vi "DDS.vi"() -> ()   [LabVIEW 2021]
uses:
  <vilib>/RTI DDS Toolkit/Types/RTI DDS Advanced Writer Configuration.ctl
  <vilib>/RTI DDS Toolkit/Types/RTI DDS Advanced Reader Configuration.ctl
  <vilib>/RTI DDS Toolkit/VIs/AdvancedCreateReader_NumI32.vi
  <vilib>/RTI DDS Toolkit/VIs/AdvancedCreateWriter_NumI32.vi
  <vilib>/RTI DDS Toolkit/VIs/Read_NumI32.vi
  <vilib>/RTI DDS Toolkit/VIs/Write_NumI32.vi
  <vilib>/RTI DDS Toolkit/Library/LVDDS_library.lvlib
panel:
  out "Control Time (ms)":i32
  out "Real Time (ms)":u32
  in  "Advanced Reader Configuration":T1={"typeName"="std_msgs::msg::dds_::Int32_", "keyName"="", "domainParticipantQoSProfile"="", "dataReaderQoSProfile"="", "forceArrayMapping?"=FALSE, "forceExclusiveReader?"=FALSE, "forceRead? (only ExclusiveReader)"=FALSE, "forceUnboundedString?"=FALSE}
  in  "Advanced Writer Configuration":T2={"typeName"="std_msgs::msg::dds_::Int32_", "keyName"="", "domainParticipantQoSProfile"="", "dataWriterQoSProfile"="", "forceArrayMapping?"=FALSE, "forceUnboundedString?"=FALSE}
  in  "stop":bool
  # "DDS"
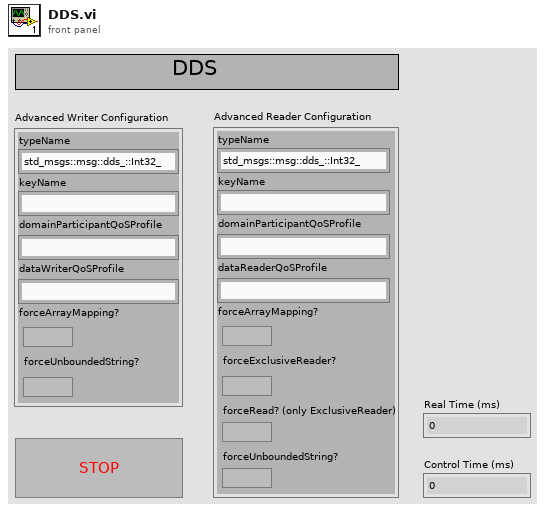
[diagram p1: front panel]
types:
  T1 = typedef "LVDDS_library.lvlib/RTI DDS Advanced Reader Configuration.ctl" = cluster{"typeName":string, "keyName":string, "domainParticipantQoSProfile":string, "dataReaderQoSProfile":string, "forceArrayMapping?":bool, "forceExclusiveReader?":bool, "forceRead? (only ExclusiveReader)":bool, "forceUnboundedString?":bool}
  T2 = typedef "LVDDS_library.lvlib/RTI DDS Advanced Writer Configuration.ctl" = cluster{"typeName":string, "keyName":string, "domainParticipantQoSProfile":string, "dataWriterQoSProfile":string, "forceArrayMapping?":bool, "forceUnboundedString?":bool}
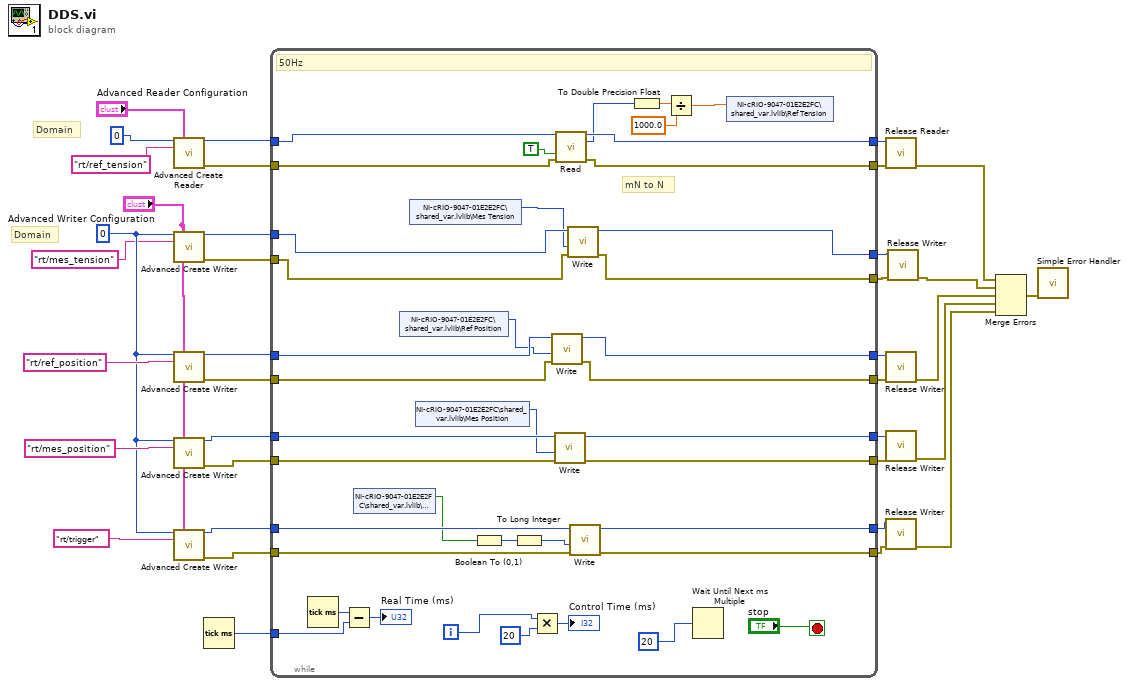
[diagram p0: block diagram]
diagram:
  w4 = u32 0 ("Domain Id")
  # "Domain"
  # "Domain"
  n1 = call-poly <vilib>:"Advanced Create Reader.vi"("Domain Id"=u32 0, "Advanced Reader Configuration"="Advanced Reader Configuration", "Topic Name"="rt/ref_tension") -> ("DDS Object Ref"=w20:u64, "error out"=w21:errorcluster)  [unwired: 11 in]
  n2 = call-poly <vilib>:"Advanced Create Writer.vi"("Domain Id"=w4, "Advanced Writer Configuration"="Advanced Writer Configuration", "Topic Name"="rt/mes_tension") -> ("DDS Object Ref"=w9:u64, "error out"=w8:errorcluster)  [unwired: 11 in]
  n3 = call-poly <vilib>:"Advanced Create Writer.vi"("Domain Id"=w4, "Advanced Writer Configuration"="Advanced Writer Configuration", "Topic Name"="rt/ref_position") -> ("DDS Object Ref"=w15:u64, "error out"=w16:errorcluster)  [unwired: 11 in]
  n4 = call-poly <vilib>:"Advanced Create Writer.vi"("Domain Id"=w4, "Advanced Writer Configuration"="Advanced Writer Configuration", "Topic Name"="rt/mes_position") -> ("DDS Object Ref"=w35:u64, "error out"=w34:errorcluster)  [unwired: 11 in]
  n5 = call-poly <vilib>:"Advanced Create Writer.vi"("Domain Id"=w4, "Advanced Writer Configuration"="Advanced Writer Configuration", "Topic Name"="rt/trigger") -> ("DDS Object Ref"=w27:u64, "error out"=w28:errorcluster)  [unwired: 11 in]
  n6 = Tick Count (ms)() -> (millisecond timer value=w10:u32)
  n7 = while {
    tunnel: w10 -> [w51]
    tunnel: w27 -> [w70]
    tunnel: [w69] -> w26
    tunnel: w28 -> [w71]
    tunnel: [w68] -> w25
    tunnel: w34 -> [w74]
    tunnel: [w72] -> w32
    tunnel: w35 -> [w75]
    tunnel: [w73] -> w33
    tunnel: w16 -> [w63]
    tunnel: [w61] -> w14
    tunnel: w15 -> [w62]
    tunnel: [w60] -> w13
    tunnel: w9 -> [w46]
    tunnel: w8 -> [w45]
    tunnel: [w44] -> w7
    tunnel: [w43] -> w6
    tunnel: w21 -> [w67]
    tunnel: [w64] -> w18
    tunnel: w20 -> [w66]
    tunnel: [w65] -> w19
    i -> [w50]
    stop <- "stop" stop-if-true
    # "mN to N"
    # "50Hz"
    n8 = Tick Count (ms)() -> (millisecond timer value=w52:u32)
    n9 = Subtract(x=w52, y=w51) -> (x-y=→"Real Time (ms)":u32)
    n10 = shared-variable "NI-cRIO-9047-01E2E2FC\\shared_var.lvlib\\Trigger"() -> (w58:bool)  [unwired: 1 in, 1 out]
    n11 = shared-variable "NI-cRIO-9047-01E2E2FC\\shared_var.lvlib\\Ref Position"() -> (w37:i32)  [unwired: 1 in, 1 out]
    n12 = shared-variable "NI-cRIO-9047-01E2E2FC\\shared_var.lvlib\\Mes Tension"() -> (w42:i32)  [unwired: 1 in, 1 out]
    n13 = shared-variable "NI-cRIO-9047-01E2E2FC\\shared_var.lvlib\\Mes Position"() -> (w55:i32)  [unwired: 1 in, 1 out]
    n14 = Boolean To (0,1)(Boolean=w58) -> (0, 1=w57:i16)
    n15 = To Long Integer(number=w57) -> (32bit integer=w56:i32)
    n16 = Multiply(x=w50, y=20) -> (x*y=→"Control Time (ms)":i32)
    n17 = call-poly <vilib>:"Write.vi"("error in (no error)"=w63, "Data"=w37, "DDS Object Ref in"=w62) -> ("error out"=w61:errorcluster, "DDS Object Ref out"=w60:u64)  [unwired: 7 in]
    n18 = call-poly <vilib>:"Write.vi"("error in (no error)"=w74, "Data"=w55, "DDS Object Ref in"=w75) -> ("error out"=w72:errorcluster, "DDS Object Ref out"=w73:u64)  [unwired: 7 in]
    n19 = call-poly <vilib>:"Read.vi"("DDS Object Ref in"=w66, "Only New Samples"=TRUE, "error in (no error)"=w67) -> ("DDS Object Ref out"=w65:u64, "Data"=w40:i32, "error out"=w64:errorcluster)  [unwired: 8 in, 2 out]
    n20 = call-poly <vilib>:"Write.vi"("error in (no error)"=w45, "Data"=w42, "DDS Object Ref in"=w46) -> ("error out"=w43:errorcluster, "DDS Object Ref out"=w44:u64)  [unwired: 7 in]
    n21 = call-poly <vilib>:"Write.vi"("error in (no error)"=w71, "Data"=w56, "DDS Object Ref in"=w70) -> ("error out"=w68:errorcluster, "DDS Object Ref out"=w69:u64)  [unwired: 7 in]
    n22 = To Double Precision Float(number=w40) -> (double precision float=w39:dbl)
    n23 = Divide(x=w39, y=1000.0) -> (x/y=w38:dbl)
    n24 = Wait Until Next ms Multiple(millisecond multiple=u32 20) -> ()  [unwired: 1 out]
    n25 = shared-variable "NI-cRIO-9047-01E2E2FC\\shared_var.lvlib\\Ref Tension"(w38) -> ()  [unwired: 1 in, 1 out]
  }
  n26 = call <vilib>:"Release Reader.vi"("error in (no error)"=w18, "DDS Object Ref"=w19) -> ("error out"=w1:errorcluster)  [unwired: 9 in]
  n27 = call <vilib>:"Release Writer.vi"("error in (no error)"=w14, "DDS Object Ref"=w13) -> ("error out"=w12:errorcluster)  [unwired: 9 in]
  n28 = call <vilib>:"Release Writer.vi"("error in (no error)"=w32, "DDS Object Ref"=w33) -> ("error out"=w31:errorcluster)  [unwired: 9 in]
  n29 = call <vilib>:"Release Writer.vi"("error in (no error)"=w25, "DDS Object Ref"=w26) -> ("error out"=w17:errorcluster)  [unwired: 9 in]
  n30 = call <vilib>:"Release Writer.vi"("error in (no error)"=w6, "DDS Object Ref"=w7) -> ("error out"=w2:errorcluster)  [unwired: 9 in]
  n31 = Merge Errors(w1, w2, w12, w31, w17) -> (w30:errorcluster)
  n32 = call <vilib>:"Simple Error Handler.vi"("error in (no error)"=w30) -> ()  [unwired: 4 in, 5 out]
